vi "CANOpen_ReadWrite Bidirectional Data.vi"(8 "error in":errorcluster, 9 "Hardware Output FIFO":refnum<k33>, 10 "Hardware Input FIFO":refnum<k33>, 11 "Channel Pairs":T2 {"Chan Refs" format="%.0x"}) -> (0 "error out":errorcluster, 2 "Read Occured":bool, 3 "Channel Pairs Out":T2 {"Chan Refs" format="%.0x"})   [LabVIEW 2013]
uses:
  <vilib>/NI Veristand/Custom Device API/Data Reference.ctl
  <vilib>/NI Veristand/Custom Device API/Global Data Refs.vi
  <vilib>/NI Veristand/Custom Device API/Custom Device API.lvlib
  Debug/SubVIs/Global debug.vi
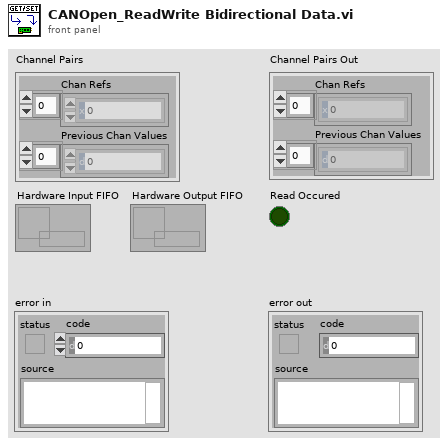
[diagram p1: front panel]
types:
  T1 = typedef "Custom Device API.lvlib/Data Reference.ctl" = i32
  T2 = cluster{"Chan Refs":T1[], "Previous Chan Values":dbl[]}
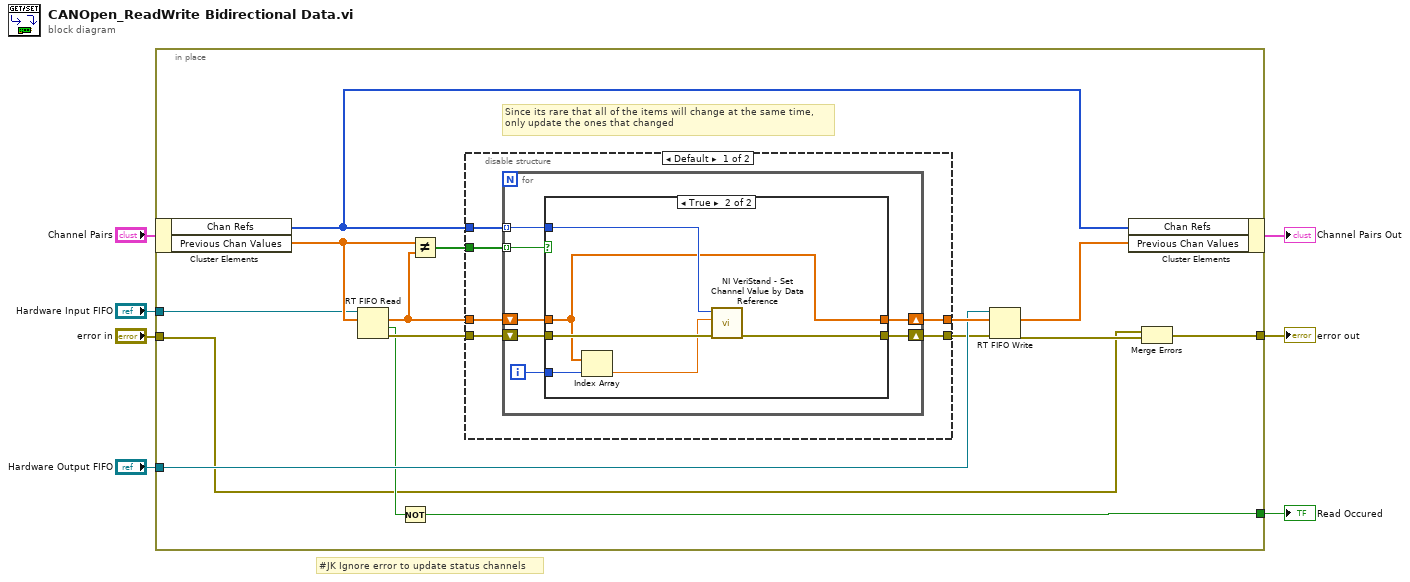
[diagram p0: block diagram]
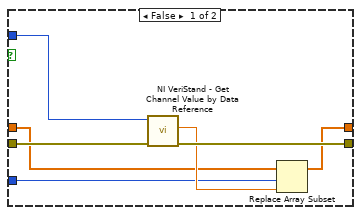
[diagram p2: hidden frame]
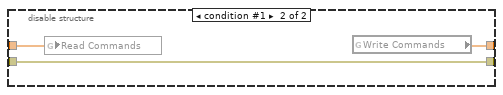
[diagram p3: hidden frame]
diagram:
  # "#JK Ignore error to update status channels"
  n1 = in-place {
    in-place-border: [w10] -> w7
    in-place-border: [w21] -> w6
    in-place-border: "error in" -> [w8]
    in-place-border: "Hardware Input FIFO" -> [w17]
    in-place-border: "Hardware Output FIFO" -> [w16]
    # "Since its rare that all of the items will change at the same time,\nonly update the ones that changed"
    n2 = in-place-cluster #1("Channel Pairs") -> ("Chan Refs"=w18:T1[], "Previous Chan Values"=w20:dbl[])
    n3 = RT FIFO Read(0:w17, 1:w20) -> (9:w13:dbl[], 10:w14:bool, 11:w15:errorcluster)  [unwired: 2 in, 2 out]
    n4 = Not(x=w14) -> (.not. x?=w21:bool)
    n5 = Not Equal?(x=w20, y=w13) -> (x != y?=w12:bool[])
    n6 = disable-structure shown="Default" {
      disable-tunnel: w15 -> [w27 w48]
      disable-tunnel: w13 -> [w26 w49]
      disable-tunnel: w18 -> [w25 _]
      disable-tunnel: w12 -> [w24 _]
      disable-tunnel: [w23 w48] -> w11
      disable-tunnel: [w22 w50] -> w19
      frame condition #0 (active) {
        n7 = for {
          shift-right: [w34] -> w23
          shift-left: w27 -> [w33]
          tunnel: w24 -> [w30] mode=indexing
          tunnel: w25 -> [w31] mode=indexing
          shift-right: [w28] -> w22
          shift-left: w26 -> [w32]
          i -> [w29]
          n8 = case shown="True" w30 {
            tunnel: w32 -> [w36 w42]
            tunnel: [w39 w46] -> w34
            tunnel: w33 -> [w40 w47]
            tunnel: w31 -> [w41 w45]
            tunnel: w29 -> [w37 w44]
            tunnel: [w35 w42] -> w28
            frame False {
              n9 = call <vilib>:"NI VeriStand - Get Channel Value by Data Reference.vi"("error in (no error)"=w40, "Data Reference in"=w41) -> ("error out"=w39:errorcluster, "Value"=w38:dbl)  [unwired: 8 in]
              n10 = Replace Array Subset(array=w36, new element=w38, index=w37) -> (w35:dbl[])
            }
            frame True {
              n11 = Index Array(array=w42, index=w44) -> (element=w43:dbl)
              n12 = call <vilib>:"NI VeriStand - Set Channel Value by Data Reference.vi"("error in (no error)"=w47, "Value"=w43, "Data Reference in"=w45) -> ("error out"=w46:errorcluster)  [unwired: 8 in]
            }
          }
        }
      }
      frame condition #1 {
        n13 = global write "Global debug.vi" "Read Commands"(w49) -> ()
        n14 = global read "Global debug.vi" "Write Commands"() -> (w50:dbl[])
      }
    }
    n15 = RT FIFO Write(0:w16, 1:w19, 3:w11) -> (11:w9:errorcluster)  [unwired: 2 in, 3 out]
    n16 = in-place-cluster #1("Chan Refs"=w18, "Previous Chan Values"=w19) -> (→"Channel Pairs Out":T2)
    n17 = Merge Errors(w8, w9) -> (w10:errorcluster)
  }
  "error out" <- w7
  "Read Occured" <- w6
